vi "Global 1.vi"() -> ()   [LabVIEW 2024]
panel:
  out "Test Log control":refnum<vi>
  in  "Test report comments":string
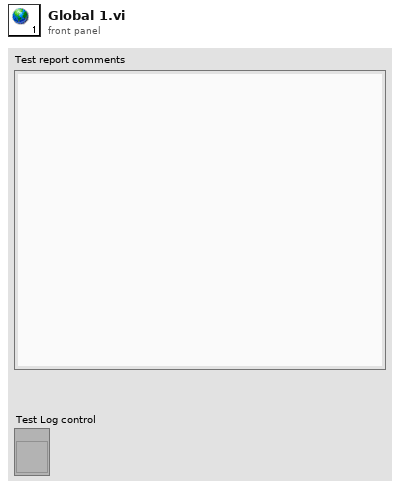
[diagram p1: front panel]
diagram:
